vi "Quiz3_TP059851_Sim Yoke Shin_Server.vi"() -> ()   [LabVIEW 2020]
uses:
  <vilib>/regexp/Match Regular Expression.xnode
panel:
  in  "Tab Control":enum32{"Page 1", "Page 2"}(tab)
  out "X / Y":dbl
  out "X x Y":dbl
  out "X - Y":dbl
  out "X + Y":dbl
  # "Server"
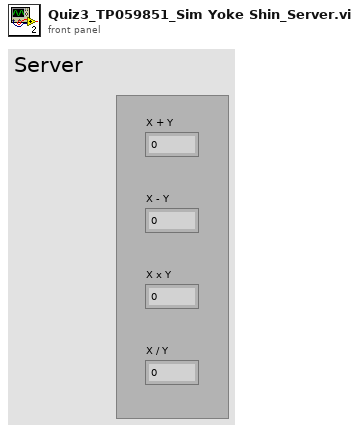
[diagram p1: front panel]
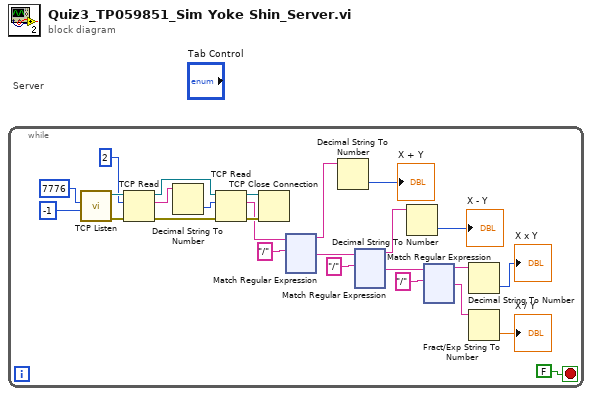
[diagram p0: block diagram]
diagram:
  # "Server"
  n1 = while {
    stop <- FALSE stop-if-true
    n2 = call <vilib>:"TCP Listen.vi"("timeout ms (wait forever: -1)"=-1, "port"=u16 7776) -> ("error out"=w21:errorcluster, "connection ID"=w25:refnum<k5>)  [unwired: 5 in, 3 out]
    n3 = TCP Read(connection ID=w25, bytes to read=2, error in (no error)=w21) -> (connection ID out=w24:refnum<k5>, data out=w17:string, error out=w20:errorcluster)  [unwired: 2 in]
    n4 = Decimal String To Number(string=w17) -> (number=w16:i32)  [unwired: 2 in, 1 out]
    n5 = TCP Read(connection ID=w24, bytes to read=w16, error in (no error)=w20) -> (connection ID out=w26:refnum<k5>, data out=w13:string, error out=w19:errorcluster)  [unwired: 2 in]
    n6 = TCP Close Connection(connection ID=w26, error in (no error)=w19) -> ()  [unwired: 1 in, 2 out]
    n7 = xnode "Match Regular Expression"("input string"=w13, "regular expression"="/") -> ("before match"=w8:string, "after match"=w11:string)  [unwired: 4 in, 3 out]
    n8 = Decimal String To Number(string=w8) -> (number=→"X + Y":i32)  [unwired: 2 in, 1 out]
    n9 = xnode "Match Regular Expression"("input string"=w11, "regular expression"="/") -> ("before match"=w7:string, "after match"=w9:string)  [unwired: 4 in, 3 out]
    n10 = Decimal String To Number(string=w7) -> (number=→"X - Y":i32)  [unwired: 2 in, 1 out]
    n11 = xnode "Match Regular Expression"("input string"=w9, "regular expression"="/") -> ("before match"=w6:string, "after match"=w5:string)  [unwired: 4 in, 3 out]
    n12 = Decimal String To Number(string=w6) -> (number=→"X x Y":i32)  [unwired: 2 in, 1 out]
    n13 = Fract/Exp String To Number(string=w5) -> (number=→"X / Y":dbl)  [unwired: 3 in, 1 out]
  }
